vi "Write Right Joystick.vi"(8 "error in (no error)":errorcluster, 10 "Joystick":T1 {"Right" min=-1.0 max=1.0 step=0.1 scale=-1.0..1.0; "Forward" min=-1.0 max=1.0 step=0.1 scale=-1.0..1.0}, 11 "Driver in":refnum<class "Driver.lvclass">) -> (0 "error out":errorcluster, 3 "Driver out":refnum<class "Driver.lvclass">)   [LabVIEW 2014, in "Driver.lvlib" / "Driver.lvclass"]
uses:
  Driver.lvclass
  Xbox One Controller/Joystick.ctl
  Driver.lvclass/Driver.ctl
  Xbox One Controller/Xbox One Controller.lvlib
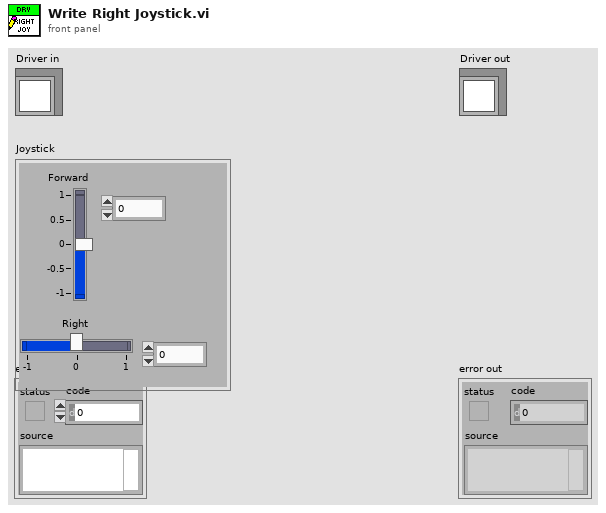
[diagram p1: front panel]
types:
  T1 = typedef "Xbox One Controller.lvlib/Joystick.ctl" = cluster{"Forward":dbl, "Right":dbl}
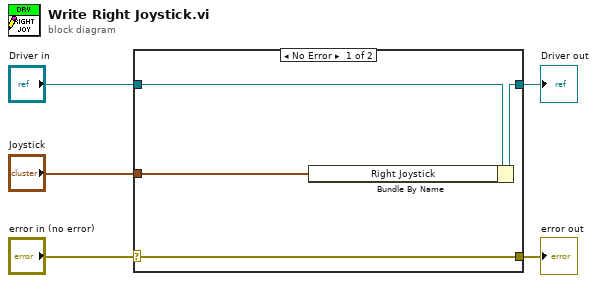
[diagram p0: block diagram]
diagram:
  n1 = case shown="No Error" "error in (no error)" {
    selector: "error in (no error)" -> [w9 w10]
    tunnel: [w9 w10] -> w4
    tunnel: [w7 w11] -> w2
    tunnel: "Driver in" -> [w8 w11]
    tunnel: "Joystick" -> [w6 _]
    frame No Error {
      n2 = Bundle By Name(cluster=w8, "Right Joystick"=w6) -> (w7:refnum<class "Driver.lvclass">)
    }
    frame Error {
    }
  }
  "error out" <- w4
  "Driver out" <- w2
